vi "5.7.5-Midbrain-Where-UDPClient.vi"() -> ()   [LabVIEW 2010]
doc: "This VI implements a client for the Named Service UDP Server.vi.\nIt connects to a service by specifying the server address and the name of the service. After sending a 'Hello' string to the server, the client receives the string sent by the server, displays the string and closes the connection.\n\n<b>Note:</b> This VI is built to work with the Named Service UDP Server.vi in UDP.llb."
uses:
  4-High Neurons/4.2-Where Sensor Typedef.ctl
  4-High Neurons/Current GPS Data.ctl
  3-Midbrain/3.2-Where/_typedefs/3.2.1-VectorNav Data.ctl
  5.0-Global.vi
panel:
  out "data":T1 {"4.2.2- Current GPS Data"."Longitude (dd.mmmmmm)" format="%#.6g"; "4.2.2- Current GPS Data"."Lattitude (dd.mmmmmm)" format="%#.6g"}
  out "String":string
  out "error out":errorcluster
  in  "error in":errorcluster
  # "Instructions:\n1. Open Named Service UDP Server.vi located in the same library.\n2. Follow the instructions on it's front panel.\n\nNote: This VI is built to work with the Named Service UDP Server.vi in UDP.llb."
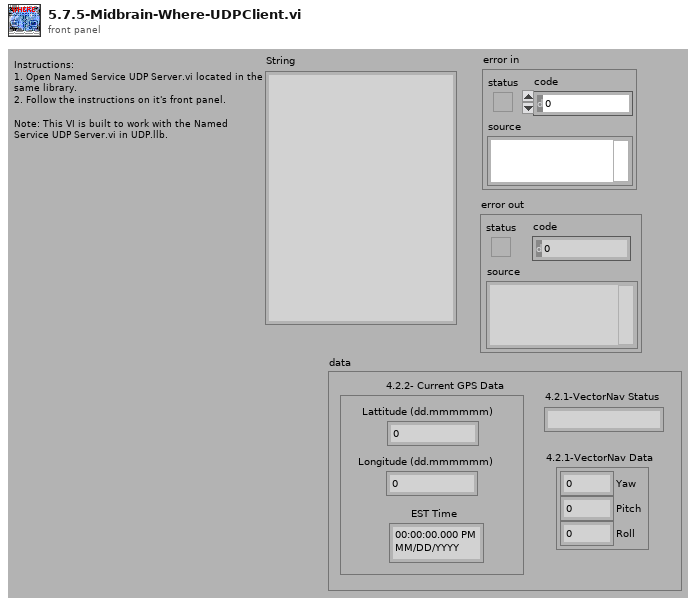
[diagram p1: front panel]
types:
  T1 = typedef "4.2-Where Sensor Typedef.ctl" = cluster{"4.2.2- Current GPS Data":T2, "4.2.1-VectorNav Data":T3, "4.2.1-VectorNav Status":string}
  T2 = typedef "Current GPS Data.ctl" = cluster{"Lattitude (dd.mmmmmm)":ext, "Longitude (dd.mmmmmm)":ext, "EST Time":timestamp}
  T3 = typedef "3.2.1-VectorNav Data.ctl" = cluster{"Yaw":dbl, "Pitch":dbl, "Roll":dbl}
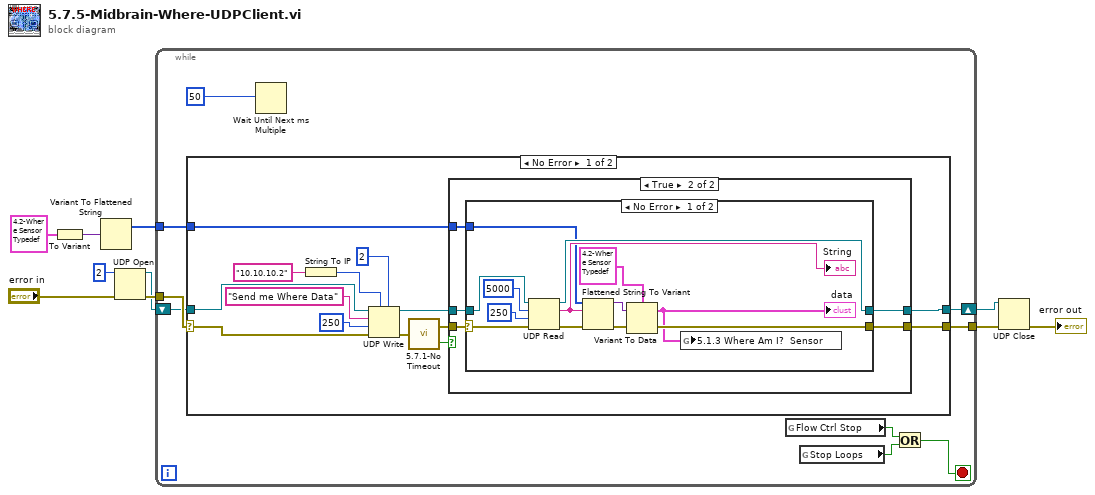
[diagram p0: block diagram]
diagram:
  n1 = To Variant(anything=T1 {"4.2.2- Current GPS Data"={"Lattitude (dd.mmmmmm)"=0.0, "Longitude (dd.mmmmmm)"=0.0, "EST Time"=timestamp(0 s since 1904-01-01)}, "4.2.1-VectorNav Data"={"Yaw"=0.0, "Pitch"=0.0, "Roll"=0.0}, "4.2.1-VectorNav Status"=""} ("Consolidated Where Data")) -> (Variant=w2:variant)
  n2 = Variant To Flattened String(Variant=w2) -> (1:w4:i16[])  [unwired: 1 out]
  n3 = UDP Open(8:"error in", 11:u16 2 ("port")) -> (port=w8:refnum<k16>, 0:w9:errorcluster)  [unwired: 3 in, 1 out]
  n4 = while {
    tunnel: [w19] -> w6
    tunnel: w9 -> [w18]
    shift-right: [w16] -> w7
    shift-left: w8 -> [w17]
    tunnel: w4 -> [w15]
    stop <- w11 stop-if-true
    n5 = case shown="No Error" w18 {
      selector: w18 -> [w33 w57]
      tunnel: [w28 w57] -> w19
      tunnel: w17 -> [w32 w56]
      tunnel: [w27 w56] -> w16
      tunnel: w15 -> [w22 _]
      frame No Error {
        n6 = String To IP(1:"10.10.10.2" ("Forbrain IP")) -> (0:w31:u32)
        n7 = UDP Write(address=w31, port or service name=u16 2, connection ID=w32, data in="Send me Where Data", 8:w33, 9:250 ("timeout ms (25000)")) -> (error out=w26:errorcluster, 3:w29:refnum<k16>)
        n8 = call "5.7.1-No Timeout.vi"("error in (no error)"=w26) -> ("No Timeout"=w24:bool, "error out"=w25:errorcluster)
        n9 = case shown="True" w24 {
          tunnel: w25 -> [w35 w40]
          tunnel: w29 -> [w34 w39]
          tunnel: [w34 w38] -> w27
          tunnel: [w35 w37] -> w28
          tunnel: w22 -> [_ w36]
          frame False {
          }
          frame True {
            n10 = case shown="No Error" w40 {
              selector: w40 -> [w53 w54]
              tunnel: w39 -> [w52 w55]
              tunnel: [w50 w55] -> w38
              tunnel: [w44 w54] -> w37
              tunnel: w36 -> [w48 _]
              frame No Error {
                n11 = UDP Read(connection ID=w52, max size (548)=5000, timeout ms (25000)=250, 8:w53) -> (data out=w49:string, error out=w45:errorcluster, 3:w50:refnum<k16>)  [unwired: 2 out]
                "String" <- w49
                n12 = Flattened String To Variant(4:w45, 6:w49, 7:w48) -> (0:w46:errorcluster, 3:w47:variant)
                n13 = Variant To Data(error in=w46, Variant=w47, type=T1 {"4.2.2- Current GPS Data"={"Lattitude (dd.mmmmmm)"=0.0, "Longitude (dd.mmmmmm)"=0.0, "EST Time"=timestamp(0 s since 1904-01-01)}, "4.2.1-VectorNav Data"={"Yaw"=0.0, "Pitch"=0.0, "Roll"=0.0}, "4.2.1-VectorNav Status"=""} ("Consolidated Where Data")) -> (error out=w44:errorcluster, data=w42:T1)
                "data" <- w42
                n14 = global write "5.0-Global.vi" "5.1.3 Where Am I?  Sensor"(w42) -> ()
              }
              frame Error {
              }
            }
          }
        }
      }
      frame Error {
      }
    }
    n15 = Wait Until Next ms Multiple(millisecond multiple=u32 50) -> ()  [unwired: 1 out]
    n16 = global read "5.0-Global.vi" "Flow Ctrl Stop"() -> (w13:bool)
    n17 = global read "5.0-Global.vi" "Stop Loops"() -> (w12:bool)
    n18 = Or(x=w13, y=w12) -> (x .or. y?=w11:bool)
  }
  n19 = UDP Close(connection ID=w7, 8:w6) -> (error out=→"error out":errorcluster)  [unwired: 1 out]
